vi "Read DIO Mode.vi"(8 "error in":errorcluster, 11 "PWM Mode in":refnum<class "PWM Mode.lvclass">) -> (0 "error out":errorcluster, 2 "DIO mode":u32, 3 "PWM Mode out":refnum<class "PWM Mode.lvclass">)   [LabVIEW 2017, in "Scan Engine Scripting.lvlib" / "PWM Mode.lvclass"]
uses:
  PWM Mode.lvclass
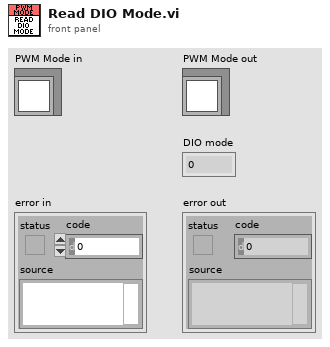
[diagram p1: front panel]
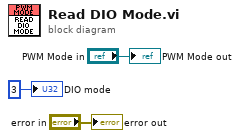
[diagram p0: block diagram]
diagram:
  "error out" <- "error in"
  "PWM Mode out" <- "PWM Mode in"
  "DIO mode" <- u32 3 ("DIO mode")
